vi "Open.vi"(8 "error in (no error)":errorcluster, 10 "INI Path":path) -> (0 "error out":errorcluster, 3 "INI Serializer out":refnum<class "INI Serializer.lvclass">)   [LabVIEW 2014, in "INI Serializer.lvclass"]
uses:
  INI Serializer.lvclass
  INI Serializer.lvclass/INI Serializer.ctl
  <vilib>/Utility/config.llb/NI_LVConfig.lvlib
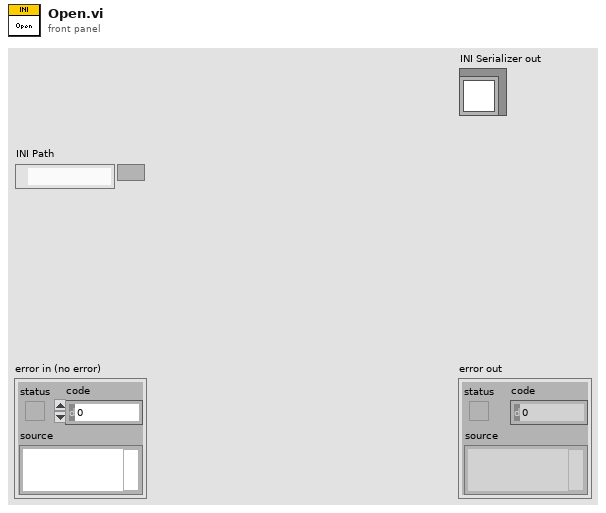
[diagram p1: front panel]
types:
  T1 = typedef "NI_LVConfig.lvlib/Config Data RefNum.ctl" = refnum<k1>
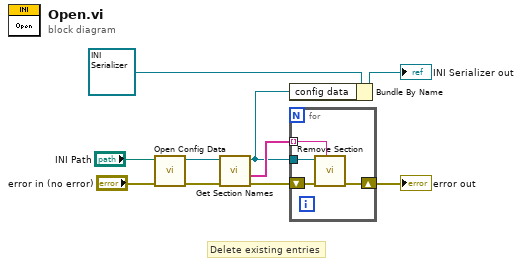
[diagram p0: block diagram]
diagram:
  # "Delete existing entries"
  n1 = call <vilib>:"Open Config Data.vi"("error in (no error)"="error in (no error)", "configuration file path"="INI Path") -> ("error out"=w4:errorcluster, "refnum"=w3:T1)  [unwired: 7 in, 1 out]
  n2 = call <vilib>:"Get Section Names.vi"("error in (no error)"=w4, "refnum"=w3) -> ("error out"=w6:errorcluster, "section names"=w5:string[], "refnum out"=w2:T1)  [unwired: 7 in]
  n3 = Bundle By Name(cluster=refnum<class "INI Serializer.lvclass"> refnum ("INI Serializer in"), "config data"=w2) -> (→"INI Serializer out":refnum<class "INI Serializer.lvclass">)
  n4 = for {
    tunnel: w2 -> [w13]
    tunnel: w5 -> [w12] mode=indexing
    shift-right: [w11] -> w1
    shift-left: w6 -> [w14]
    n5 = call <vilib>:"Remove Section.vi"("section"=w12, "error in (no error)"=w14, "refnum"=w13) -> ("error out"=w11:errorcluster)  [unwired: 6 in, 2 out]
  }
  "error out" <- w1
